vi "Time2Command.vi"(10 "TimeIn":u16) -> (2 "CommandOut":u8[](array[numeric]) format="%x")   [LabVIEW 2013]
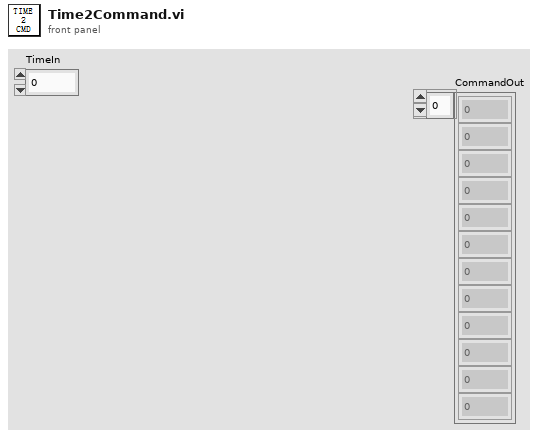
[diagram p1: front panel]
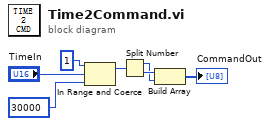
[diagram p0: block diagram]
diagram:
  n1 = In Range and Coerce(upper limit=u16 1, x="TimeIn", lower limit=u16 30000) -> (coerced(x)=w2:u16)  [unwired: 1 out]
  n2 = Split Number(x=w2) -> (hi(x)=w6:u8, lo(x)=w7:u8)
  n3 = Build Array(w7, w6) -> (→"CommandOut":u8[])
